vi "OAT Output Buffered Data (XY, N Chan).vi"(0 "XY signals":cluster{"X":dbl[], "Y":dbl[]}[](array[cluster]) {"X" format="%.2f"; "Y" format="%.2f"}, 2 "reset? (F)":bool, 7 "position info":T1, 11 "error in (no error)":errorcluster, 12 "buffer settings":T2) -> (4 "buffered XY signals":cluster{"X":dbl[], "Y":dbl[]}[](array[cluster]) {"X" format="%.2f"; "Y" format="%.2f"}, 8 "buffered position info":T1, 15 "error out":errorcluster)   [LabVIEW 2017, in "SoundVib_OAUtility.lvlib"]
doc: "Buffers the input signals and returns them in first-in first-out (FIFO) mode. Use <B>buffer settings</B> to set the buffer size and units. Each instance of this VI maintains its own state; use the N Waveforms instance of this VI to process an array of channels. Wire data to the <B>XY signal</B> input to determine the polymorphic instance to use or manually select the instance."
uses:
  <vilib>/addons/Sound and Vibration/Order Analysis/Utility/SoundVib_OAUtility.lvlib
  <vilib>/addons/Sound and Vibration/Order Analysis/Utility/SubVIs/oa_Buffer Settings.ctl
  <vilib>/addons/Sound and Vibration/Order Analysis/Misc/OAT Position Info.ctl
  <vilib>/addons/_NISVFA/_Shared subVIs/Common/svc_Get Array Subset (Index).vi
  <vilib>/addons/_NISVFA/_Shared subVIs/Common/svc_Coerce Index and Length.vi
  <vilib>/addons/_NISVFA/_Shared subVIs/Common/svc_Conditional Merge Error.vi
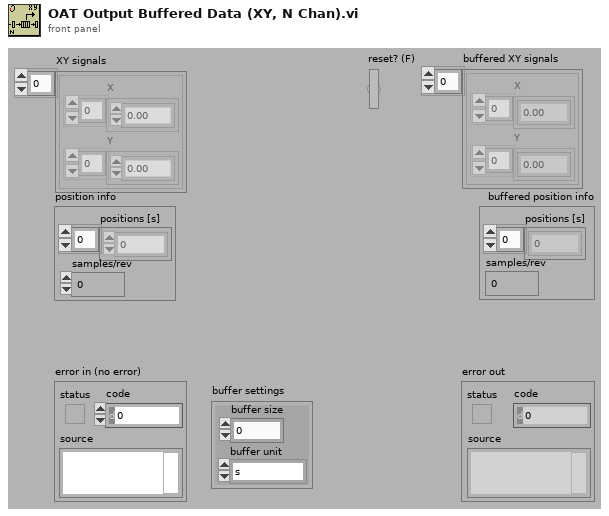
[diagram p1: front panel]
types:
  T1 = typedef "OAT Position Info.ctl" = cluster{"positions [s]":dbl[], "samples/rev":dbl}
  T2 = typedef "SoundVib_OAUtility.lvlib/oa_Buffer Settings.ctl" = cluster{"buffer size":dbl, "buffer unit":enum16{"s", "revolution", "# of samples"}}
  T3 = cluster{"positions [s]":dbl[], "samples/rev":dbl}
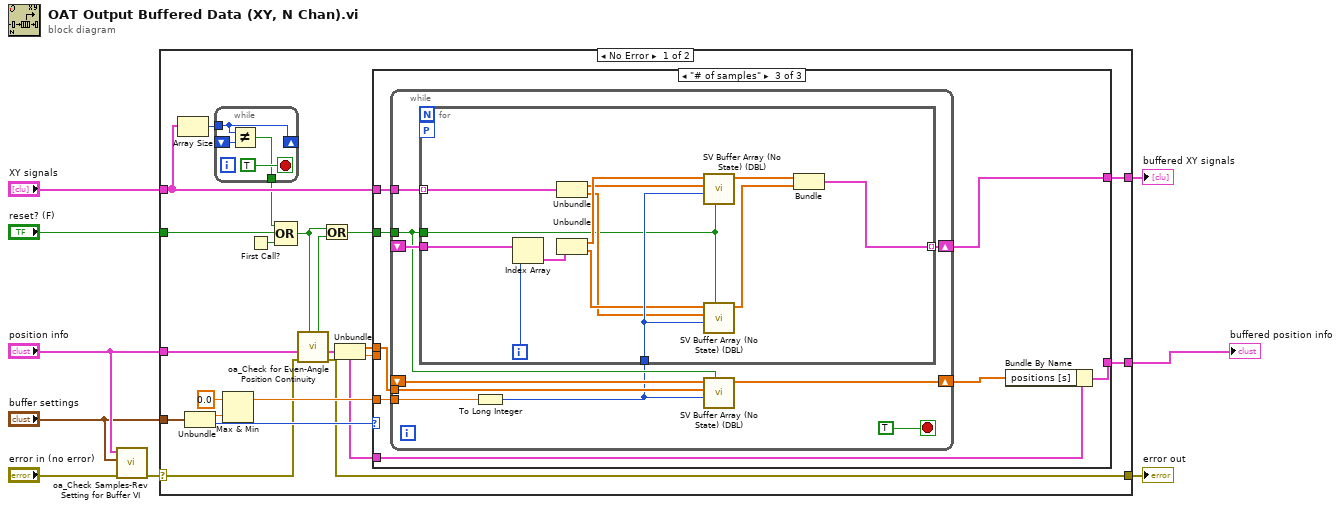
[diagram p0: block diagram]
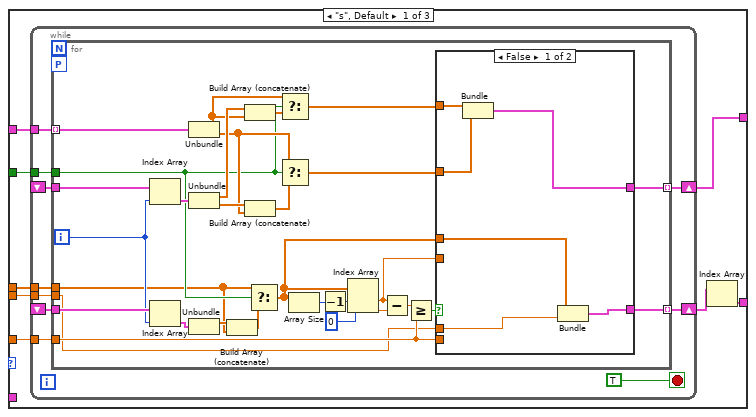
[diagram p2: hidden frame]
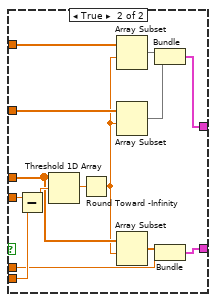
[diagram p3: hidden frame]
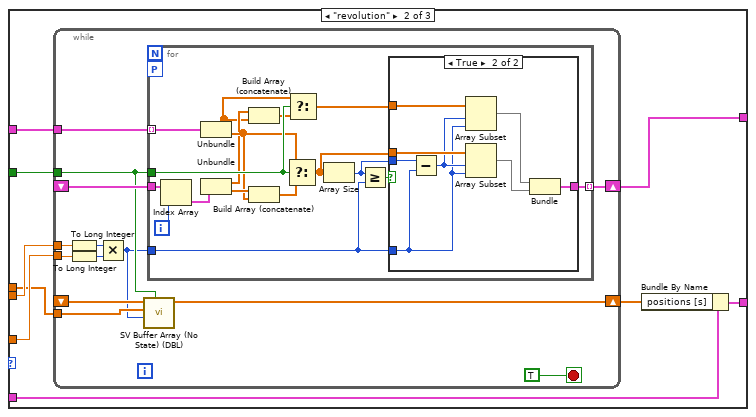
[diagram p4: hidden frame]
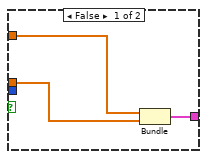
[diagram p5: hidden frame]
diagram:
  n1 = call <vilib>:"oa_Check Samples-Rev Setting for Buffer VI.vi"("error in (no error)"="error in (no error)", "buffer settings"="buffer settings", "position info"="position info") -> ("error out"=w5:errorcluster)  [unwired: 8 in]
  n2 = case shown="No Error" w5 {
    selector: w5 -> [w16 w184]
    tunnel: [w15 w184] -> w7
    tunnel: "buffer settings" -> [w30 _]
    tunnel: "XY signals" -> [w24 _]
    tunnel: "reset? (F)" -> [w21 _]
    tunnel: [w27 _] -> w6
    tunnel: "position info" -> [w19 _]
    tunnel: [w11 _] -> w1
    frame No Error {
      n3 = Array Size(array=w24) -> (size(s)=w23:i32)
      n4 = Unbundle(w30) -> ("buffer size"=w25:dbl, "buffer unit"=w26:enum16{"s", "revolution", "# of samples"})
      n5 = while {
        tunnel: w23 -> [w33]
        shift-right: [w33] -> _
        shift-left: _ -> [w34]
        tunnel: [w31] -> w22
        stop <- TRUE stop-if-true
        n6 = Not Equal?(x=w33, y=w34) -> (x != y?=w31:bool)
      }
      n7 = Max & Min(x=0.0, y=w25) -> (max(x,y)=w28:dbl)  [unwired: 1 out]
      n8 = First Call?() -> (First Call?: T/F=w20:bool)
      n9 = Compound Arithmetic op=OR(w22, w21, w20) -> (w14:bool)
      n10 = call <vilib>:"oa_Check for Even-Angle Position Continuity.vi"("reset in"=w14, "error in (no error)"=w16, "even-angle position info"=w19) -> ("error out"=w15:errorcluster, "even-angle position info dup"=w10:T1, "position not continuous"=w12:bool)  [unwired: 6 in]
      n11 = Or(x=w14, y=w12) -> (x .or. y?=w13:bool)
      n12 = Unbundle(w10) -> ("positions [s]"=w17:dbl[], "samples/rev"=w18:dbl)
      n13 = case shown="\"# of samples\"" w26 {
        tunnel: w28 -> [w41 w109 w158]
        tunnel: w24 -> [w40 w111 w160]
        tunnel: w13 -> [w39 w110 w159]
        tunnel: [w38 w103 w157] -> w27
        tunnel: w17 -> [w42 w107 w156]
        tunnel: w18 -> [w35 w108 _]
        tunnel: [w36 w104 w153] -> w11
        tunnel: w10 -> [_ w106 w155]
        frame "s", Default {
          n14 = while {
            tunnel: w42 -> [w50]
            tunnel: w41 -> [w49]
            tunnel: w40 -> [w47]
            shift-right: [w52] -> w38
            shift-left: _ -> [w48]
            tunnel: w39 -> [w46]
            shift-right: [w45] -> w37
            shift-left: _ -> [w44]
            tunnel: w35 -> [w43]
            stop <- TRUE stop-if-true
            n15 = for {
              tunnel: [w76] -> w52 mode=indexing
              tunnel: w50 -> [w55]
              tunnel: w49 -> [w74]
              tunnel: w48 -> [w64]
              tunnel: w47 -> [w67] mode=indexing
              tunnel: w46 -> [w58]
              tunnel: [w62] -> w45 mode=indexing
              tunnel: w44 -> [w61]
              tunnel: w43 -> [w53]
              workers-P: _ -> [_]
              i -> [w60]
              n16 = Index Array(array=w64, index=w60) -> (element=w63:cluster{"X":dbl[], "Y":dbl[]})
              n17 = Index Array(array=w61, index=w60) -> (element=w57:T3)
              n18 = Unbundle(w67) -> ("X"=w72:dbl[], "Y"=w69:dbl[])
              n19 = Unbundle(w63) -> ("X"=w73:dbl[], "Y"=w70:dbl[])
              n20 = Unbundle(w57) -> ("positions [s]"=w56:dbl[])  [unwired: 1 out]
              n21 = Build Array (concatenate)(w56, w55) -> (w54:dbl[])
              n22 = Build Array (concatenate)(w73, w72) -> (w71:dbl[])
              n23 = Build Array (concatenate)(w70, w69) -> (w68:dbl[])
              n24 = Select(t=w55, s=w58, f=w54) -> (s? t:f=w59:dbl[])
              n25 = Select(t=w72, s=w58, f=w71) -> (s? t:f=w66:dbl[])
              n26 = Select(t=w69, s=w58, f=w68) -> (s? t:f=w65:dbl[])
              n27 = Array Size(array=w59) -> (size(s)=w82:i32)
              n28 = Decrement(x=w82) -> (x-1=w81:i32)
              n29 = Index Array(array=w59, index #1=w81, index #2=0 ("index")) -> (element #1=w75:dbl, element #2=w79:dbl)
              n30 = Subtract(x=w75, y=w79) -> (x-y=w78:dbl)
              n31 = Greater Or Equal?(x=w78, y=w74) -> (x >= y?=w77:bool)
              n32 = case shown="False" w77 {
                tunnel: [w88 w96] -> w76
                tunnel: w59 -> [w85 w93]
                tunnel: w75 -> [_ w102]
                tunnel: w74 -> [_ w101]
                tunnel: w66 -> [w87 w95]
                tunnel: w65 -> [w86 w94]
                tunnel: [w84 w91] -> w62
                tunnel: w53 -> [w83 w89]
                frame False {
                  n33 = Bundle("X"=w87, "Y"=w86) -> (w88:cluster{"X":dbl[], "Y":dbl[]})  [unwired: 1 in]
                  n34 = Bundle("positions [s]"=w85, "samples/rev"=w83) -> (w84:T3)  [unwired: 1 in]
                }
                frame True {
                  n35 = Subtract(x=w102, y=w101) -> (x-y=w100:dbl)
                  n36 = Threshold 1D Array(2:w100, 3:w93) -> (0:w99:dbl)  [unwired: 1 in]
                  n37 = Round Toward -Infinity(1:w99) -> (0:w90:dbl)
                  n38 = Array Subset(array=w95, index=w90) -> (w98:dbl[])  [unwired: 1 in]
                  n39 = Array Subset(array=w94, index=w90) -> (w97:dbl[])  [unwired: 1 in]
                  n40 = Array Subset(array=w93, index=w90) -> (w92:dbl[])  [unwired: 1 in]
                  n41 = Bundle(w98, w97) -> (w96:cluster{dbl[], dbl[]})  [unwired: 1 in]
                  n42 = Bundle(w92, "samples/rev"=w89) -> (w91:cluster{dbl[], "samples/rev":dbl})  [unwired: 1 in]
                }
              }
            }
          }
          n43 = Index Array(array=w37) -> (element=w36:T3)  [unwired: 1 in]
        }
        frame "revolution" {
          n44 = while {
            tunnel: w111 -> [w124]
            shift-right: [w122] -> w103
            shift-left: _ -> [w121]
            tunnel: w110 -> [w114]
            tunnel: w109 -> [w117]
            tunnel: w108 -> [w118]
            shift-right: [w112] -> w105
            shift-left: _ -> [w116]
            tunnel: w107 -> [w115]
            stop <- TRUE stop-if-true
            n45 = To Long Integer(number=w118) -> (32bit integer=w120:i32)
            n46 = To Long Integer(number=w117) -> (32bit integer=w119:i32)
            n47 = Multiply(x=w120, y=w119) -> (x*y=w113:i32)
            n48 = call <vilib>:"SV Buffer Array (No State) (DBL).vi"("clear buffer (False)"=w114, "buffer length  [samples] (-1 = unlimited)"=w113, "Y"=w115, "buffer in"=w116) -> ("buffer out"=w112:dbl[])  [unwired: 7 in]
            n49 = for {
              tunnel: w124 -> [w141] mode=indexing
              tunnel: w114 -> [w138]
              tunnel: [w136] -> w122 mode=indexing
              tunnel: w121 -> [w128]
              tunnel: w113 -> [w125]
              workers-P: _ -> [_]
              i -> [w127]
              n50 = Index Array(array=w128, index=w127) -> (element=w126:cluster{"X":dbl[], "Y":dbl[]})
              n51 = Unbundle(w141) -> ("X"=w129:dbl[], "Y"=w133:dbl[])
              n52 = Unbundle(w126) -> ("X"=w130:dbl[], "Y"=w134:dbl[])
              n53 = Build Array (concatenate)(w130, w129) -> (w131:dbl[])
              n54 = Build Array (concatenate)(w134, w133) -> (w132:dbl[])
              n55 = Select(t=w133, s=w138, f=w132) -> (s? t:f=w140:dbl[])
              n56 = Select(t=w129, s=w138, f=w131) -> (s? t:f=w137:dbl[])
              n57 = Array Size(array=w140) -> (size(s)=w139:i32)
              n58 = Greater Or Equal?(x=w139, y=w125) -> (x >= y?=w135:bool)
              n59 = case shown="True" w135 {
                tunnel: w140 -> [w142 w150]
                tunnel: w139 -> [_ w149]
                tunnel: w137 -> [w143 w151]
                tunnel: [w144 w152] -> w136
                tunnel: w125 -> [_ w145]
                frame False {
                  n60 = Bundle("X"=w143, "Y"=w142) -> (w144:cluster{"X":dbl[], "Y":dbl[]})  [unwired: 1 in]
                }
                frame True {
                  n61 = Subtract(x=w149, y=w145) -> (x-y=w148:i32)
                  n62 = Array Subset(array=w151, index=w148, length=w145) -> (w146:dbl[])
                  n63 = Array Subset(array=w150, index=w148, length=w145) -> (w147:dbl[])
                  n64 = Bundle(w146, w147) -> (w152:cluster{dbl[], dbl[]})  [unwired: 1 in]
                }
              }
            }
          }
          n65 = Bundle By Name(cluster=w106, "positions [s]"=w105) -> (w104:T1)
        }
        frame "# of samples" {
          n66 = while {
            tunnel: w160 -> [w170]
            shift-right: [w168] -> w157
            shift-left: _ -> [w167]
            tunnel: w159 -> [w165]
            tunnel: w158 -> [w166]
            shift-right: [w163] -> w154
            shift-left: _ -> [w164]
            tunnel: w156 -> [w162]
            stop <- TRUE stop-if-true
            n67 = To Long Integer(number=w166) -> (32bit integer=w161:i32)
            n68 = for {
              tunnel: w170 -> [w183] mode=indexing
              tunnel: w161 -> [w178]
              tunnel: w165 -> [w171]
              tunnel: [w182] -> w168 mode=indexing
              tunnel: w167 -> [w181]
              workers-P: _ -> [_]
              i -> [w180]
              n69 = Index Array(array=w181, index=w180) -> (element=w179:cluster{"buffer out":dbl[], "buffer out":dbl[]})
              n70 = Unbundle(w183) -> ("X"=w176:dbl[], "Y"=w174:dbl[])
              n71 = Unbundle(w179) -> ("buffer out"=w177:dbl[], "buffer out"=w175:dbl[])
              n72 = call <vilib>:"SV Buffer Array (No State) (DBL).vi"("clear buffer (False)"=w171, "buffer length  [samples] (-1 = unlimited)"=w178, "Y"=w176, "buffer in"=w177) -> ("buffer out"=w173:dbl[])  [unwired: 7 in]
              n73 = call <vilib>:"SV Buffer Array (No State) (DBL).vi"("clear buffer (False)"=w171, "buffer length  [samples] (-1 = unlimited)"=w178, "Y"=w174, "buffer in"=w175) -> ("buffer out"=w172:dbl[])  [unwired: 7 in]
              n74 = Bundle("buffer out"=w173, "buffer out"=w172) -> (w182:cluster{"buffer out":dbl[], "buffer out":dbl[]})  [unwired: 1 in]
            }
            n75 = call <vilib>:"SV Buffer Array (No State) (DBL).vi"("clear buffer (False)"=w165, "buffer length  [samples] (-1 = unlimited)"=w161, "Y"=w162, "buffer in"=w164) -> ("buffer out"=w163:dbl[])  [unwired: 7 in]
          }
          n76 = Bundle By Name(cluster=w155, "positions [s]"=w154) -> (w153:T1)
        }
      }
    }
    frame Error {
    }
  }
  "error out" <- w7
  "buffered XY signals" <- w6
  "buffered position info" <- w1
